vi "Actor Core.vi"(8 "error in":errorcluster, 11 "Child Actor in":refnum<class "Child Actor.lvclass">) -> (0 "error out":errorcluster, 3 "Actor out":refnum<class "Actor.lvclass">)   [LabVIEW 2012, in "Child Actor.lvclass"]
doc: "(<B>Filename</B>: Actor Framework.lvlib:Actor.lvclass:Actor Core.vi)\n\nReceives messages to the actor, reacts to them, and initiates any error handling that may shut the actor down.\n\nDescendant classes may override this VI to append parallel tasks for the actor to complete while it handles messages. Overrides use the Call Parent Method node."
uses:
  Child Actor.lvclass
  <vilib>/ActorFramework/Actor/Actor.lvclass
  Child Actor.lvclass/Child Actor.ctl
  <vilib>/ActorFramework/Actor/Actor.lvclass/Actor.ctl
  <vilib>/ActorFramework/Message Enqueuer/Message Enqueuer.lvclass/Message Enqueuer.ctl
  Parent Actor Messages/Get State from Child Msg/Get State from Child Msg.lvclass/Get State from Child Msg.ctl
  <vilib>/ActorFramework/Message Enqueuer/Init from Existing Queue.vi
  <vilib>/ActorFramework/Message Enqueuer/Enqueue.vi
  <vilib>/ActorFramework/Message Priority Queue/Priority Enqueue.vi
  <vilib>/ActorFramework/Message Enqueuer/Message Enqueuer.lvclass
  <vilib>/ActorFramework/Stop Msg/Stop Msg.lvclass
  Parent Actor Messages/Get State from Child Msg/Get State from Child Msg.lvclass
panel:
  in  "Child Control":bool
  out "Child Indicator":bool
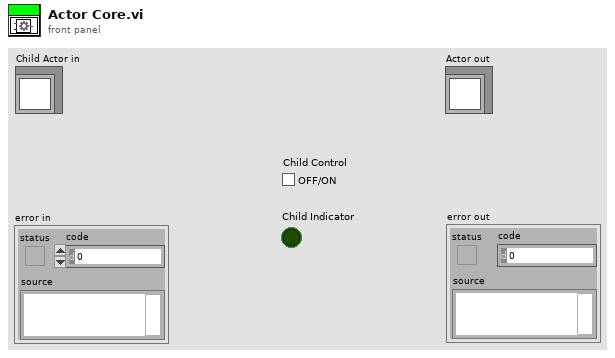
[diagram p1: front panel]
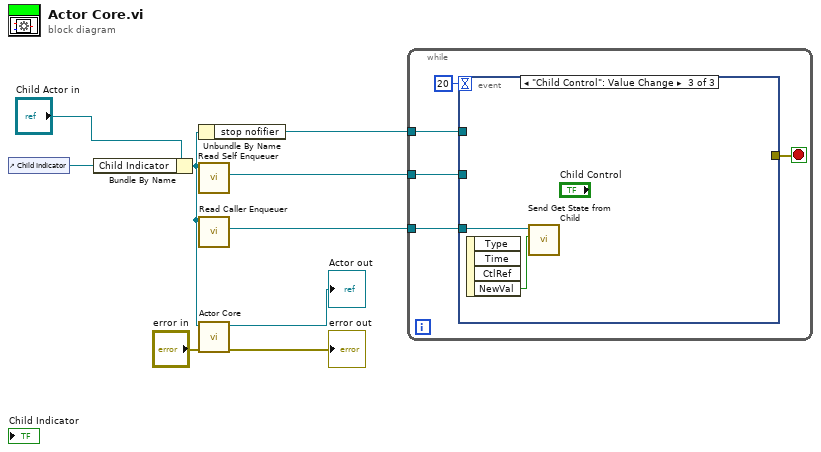
[diagram p0: block diagram]
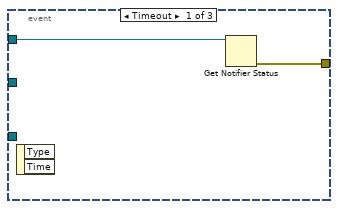
[diagram p2: hidden frame]
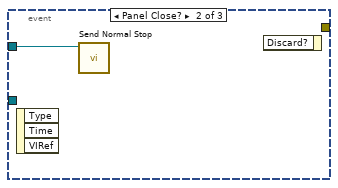
[diagram p3: hidden frame]
diagram:
  n1 = control-ref of="Child Indicator"() -> (w3:refnum<vi>)
  n2 = Bundle By Name(cluster="Child Actor in", "Child Indicator"=w3) -> (w2:refnum<class "Child Actor.lvclass">)
  n3 = Unbundle By Name(w2) -> ("stop nofifier"=w6:refnum<notifier>)
  n4 = call <vilib>:"Read Self Enqueuer.vi"("Actor"=w2) -> ("Self Enqueuer"=w5:refnum<class "Message Enqueuer.lvclass">)  [unwired: 10 in]
  n5 = call <vilib>:"Read Caller Enqueuer.vi"("Actor"=w2) -> ("Caller Enqueuer"=w1:refnum<class "Message Enqueuer.lvclass">)  [unwired: 10 in]
  n6 = call-parent "Actor Core.vi"("error in"="error in", "Actor in"=w2) -> ("error out"=→"error out":errorcluster, "Actor out"=→"Actor out":refnum<class "Actor.lvclass">)  [unwired: 8 in]
  n7 = while {
    tunnel: w6 -> [w13]
    tunnel: w5 -> [w11]
    tunnel: w1 -> [w10]
    stop <- w12 stop-if-true
    n8 = event shown="[2] \"Child Control\": Value Change" {
      selector: _ -> [_ _ _]
      dyn-events: _ -> [_ _ _]
      timeout: 20 -> [_ _ _]
      tunnel: w13 -> [w16 _ _]
      tunnel: [w15 _ _] -> w12
      tunnel: w11 -> [_ w17 _]
      tunnel: w10 -> [_ _ w18]
      event Timeout {
        n9 = event-data() -> ()  [unwired: 1 in, 2 out]
        n10 = Get Notifier Status(notifier=w16) -> (error out=w15:errorcluster)  [unwired: 1 in, 4 out]
      }
      event Panel Close? {
        n11 = event-data() -> ()  [unwired: 1 in, 3 out]
        n12 = call <vilib>:"Send Normal Stop.vi"("Message Enqueuer"=w17) -> ()  [unwired: 10 in, 1 out]
        n13 = event-data() -> ()  [unwired: 2 in, 1 out]
      }
      event "Child Control": Value Change {
        n14 = event-data() -> ("NewVal"=w19:bool)  [unwired: 1 in, 3 out]
        n15 = call "Send Get State from Child.vi"("Boolean"=w19, "Message Enqueuer"=w18) -> ()  [unwired: 8 in, 2 out]
      }
    }
  }
